vi "Test Compare Multiple Numerical Values All Inside Tolerance Passes.vi"(8 "error in (no error)":errorcluster, 11 "Test Case In":refnum<class "Tolerant Numeric Comparator Test.lvclass">) -> (0 "error out":errorcluster, 3 "Test Case Out":refnum<class "Tolerant Numeric Comparator Test.lvclass">)   [LabVIEW 2020, in "Tolerant Numeric Comparator Test.lvclass"]
uses:
  Tolerant Numeric Comparator Test.lvclass
  C:/Program Files (x86)/National Instruments/LabVIEW 2020/vi.lib/Astemes/LUnit/Test Case.lvclass
  <vilib>/Astemes/LUnit/Test Case.lvclass/Test Case.ctl
  <vilib>/Astemes/LUnit/Append Fail Result.vi
  <vilib>/Astemes/LUnit/Append Pass Result.vi
  Mock VI Call/Mock VI Call.lvclass
  C:/git/astemes-lmock/sandbox/Call/VI Call.lvclass
  Tolerant Numeric Comparator/Tolerant Numeric Comparator.lvclass
  <vilib>/Astemes/LUnit/Test Case.lvclass
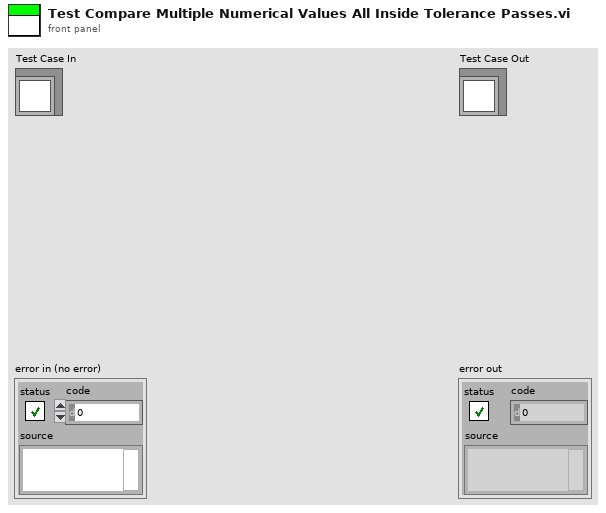
[diagram p1: front panel]
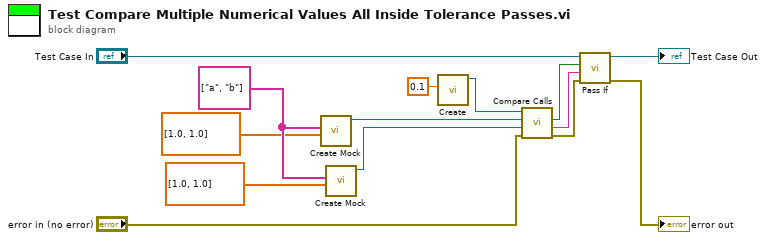
[diagram p0: block diagram]
diagram:
  w3 = string[] ["a", "b"] ("Control Label")
  n1 = call "Create Mock.vi"("Control value"=dbl[] [1.0, 1.0], "Control Label"=w3) -> ("Mock VI Call Out"=w14:refnum<class "Mock VI Call.lvclass">)  [unwired: 8 in, 1 out]
  n2 = call "Create Mock.vi"("Control value"=dbl[] [1.0, 1.0], "Control Label"=w3) -> ("Mock VI Call Out"=w13:refnum<class "Mock VI Call.lvclass">)  [unwired: 8 in, 1 out]
  n3 = call "Create.vi"("Tolerance"=0.1) -> ("Tolerant Numeric Comparator Out"=w11:refnum<class "Tolerant Numeric Comparator.lvclass">)  [unwired: 9 in, 1 out]
  n4 = call-dynamic "Compare Calls.vi"("error in (no error)"="error in (no error)", "VI Call 2"=w13, "VI Call 1"=w14, "Tolerant Numeric Comparator In"=w11) -> ("error out"=w7:errorcluster, "Description"=w4:string, "Equal?"=w5:bool)  [unwired: 5 in]
  n5 = call <vilib>:"Pass If.vi"("error in (no error)"=w7, "Message"=w4, "Pass?"=w5, "LUnit Test Case In"="Test Case In") -> ("error out"=→"error out":errorcluster, "LUnit Test Case Out"=→"Test Case Out":refnum<class "Tolerant Numeric Comparator Test.lvclass">)  [unwired: 6 in]
